vi "get Data Element.vi"(0 "LVx - Template Command in":refnum<class "LVx - Template Command.lvclass">, 11 "error in (no error)":errorcluster) -> (4 "LVx - Template Command out":refnum<class "LVx - Template Command.lvclass">, 6 "Test String":T1, 15 "error out":errorcluster)   [LabVIEW 2011, in "LVx.lvlib" / "LVx - Template Command.lvclass"]
uses:
  LVx - Template Command.lvclass
  Command Data Element.ctl
  LVx - Template Command.lvclass/LVx - Template Command.ctl
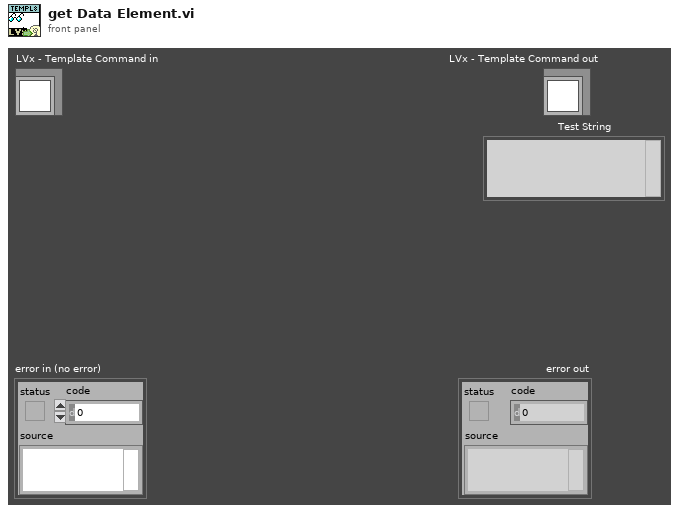
[diagram p1: front panel]
types:
  T1 = typedef "LVx.lvlib/LVx - Template Command.lvclass/Command Data Element.ctl" = string
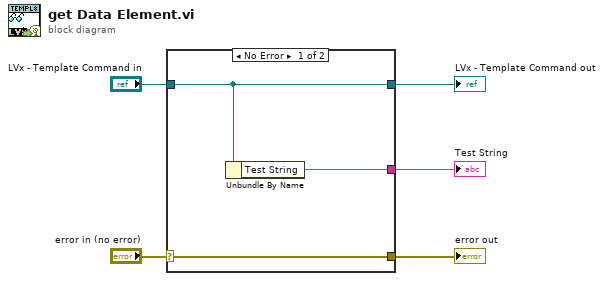
[diagram p0: block diagram]
diagram:
  n1 = case shown="No Error" "error in (no error)" {
    selector: "error in (no error)" -> [w8 w9]
    tunnel: [w8 w9] -> w4
    tunnel: [w6 w10] -> w2
    tunnel: "LVx - Template Command in" -> [w6 w10]
    tunnel: [w7 _] -> w1
    frame No Error {
      n2 = Unbundle By Name(w6) -> ("Test String"=w7:T1)
    }
    frame Error {
    }
  }
  "error out" <- w4
  "LVx - Template Command out" <- w2
  "Test String" <- w1
